vi "Change Path.vi"(8 "error in (no error)":errorcluster, 9 "Same File":bool, 10 "Path Refnum in":refnum<vi>, 11 "Path in":refnum<vi>) -> (0 "error out":errorcluster)   [LabVIEW 2020]
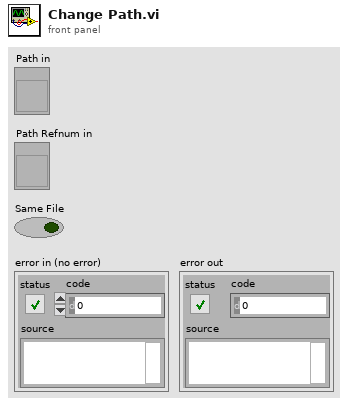
[diagram p1: front panel]
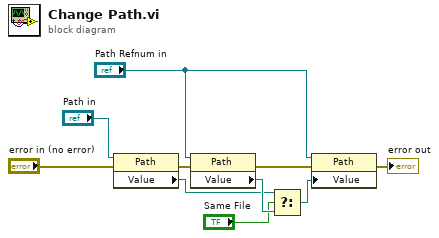
[diagram p0: block diagram]
diagram:
  n1 = property on="Property Node" class="Path"(reference="Path in", error in="error in (no error)") -> (error out=w10:errorcluster, "Value"=w5:path)  [unwired: 1 out]
  n2 = property on="Property Node" class="Path"(reference="Path Refnum in", error in=w10) -> (error out=w8:errorcluster, "Value"=w6:path)  [unwired: 1 out]
  n3 = Select(t=w5, s="Same File", f=w6) -> (s? t:f=w7:path)
  n4 = property on="Property Node" class="Path"(reference="Path Refnum in", error in=w8, "Value"=w7) -> (error out=→"error out":errorcluster)  [unwired: 1 out]
